vi "Configure.vi"(8 "error in (no error)":errorcluster, 11 "Switching Times in":refnum<class "Switching Time.lvclass">) -> (0 "error out":errorcluster, 3 "Switching Times out":refnum<class "Switching Time.lvclass">)   [LabVIEW 2020, in "Switching Time.lvclass"]
doc: "Configure the measurements paramaters to sweep.\nThis should be a pop up interface invoked by the configure test button on the main panel."
uses:
  Switching Time.lvclass
  Controls/Method.ctl
panel:
  in  "System Cancel Button":bool
  in  "Channels and optional channel names":cluster{"Enabled":bool, "Channel name":string}[](array[cluster])
  in  "Method":T1
  in  "OK Button":bool
  # "Please setup\noscilloscope\nmanually.\nE.g. vertical \nand horizontal \nrange, trigger etc."
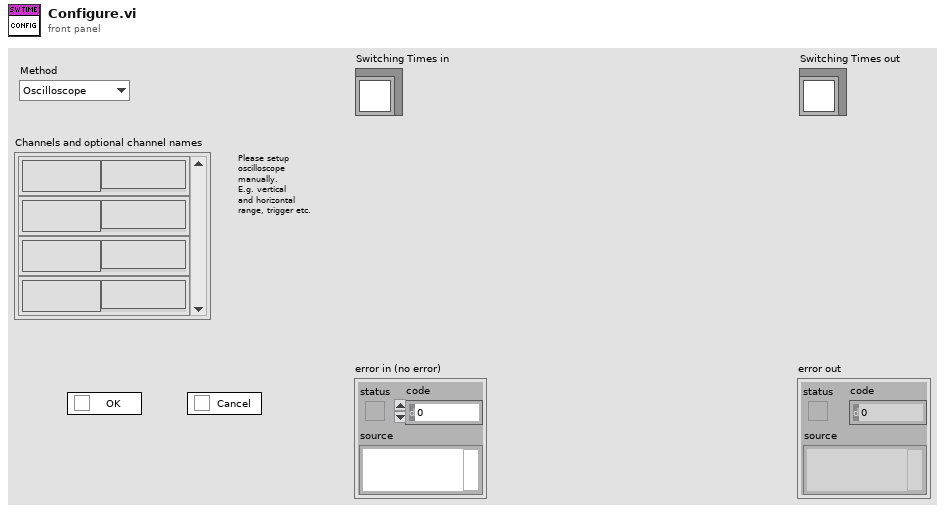
[diagram p1: front panel]
types:
  T1 = typedef "Switching Time.lvclass/Method.ctl" = enum16{"Oscilloscope", "Spectrum Analyzer"}
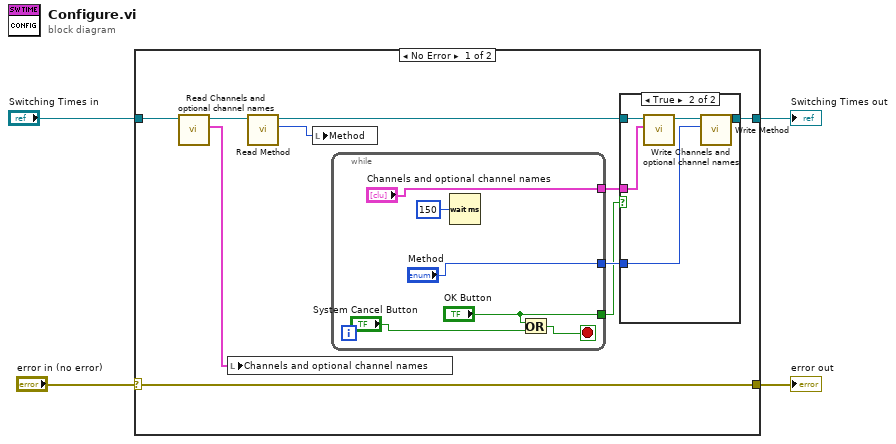
[diagram p0: block diagram]
diagram:
  n1 = case shown="No Error" "error in (no error)" {
    selector: "error in (no error)" -> [w12 w28]
    tunnel: "Switching Times in" -> [w9 w27]
    tunnel: [w14 w27] -> w2
    tunnel: [w12 w28] -> w1
    frame No Error {
      n2 = call-dynamic "Read Channels and optional channel names.vi"("Switching Time in"=w9) -> ("Channels and optional channel names"=w7:cluster{"Enabled":bool, "Channel name":string}[], "Switching Time out"=w10:refnum<class "Switching Time.lvclass">)  [unwired: 9 in]
      n3 = local write "Channels and optional channel names"(w7) -> ()
      n4 = call-dynamic "Read Method.vi"("Switching Time in"=w10) -> ("Method"=w6:T1, "Switching Time out"=w8:refnum<class "Switching Time.lvclass">)  [unwired: 9 in]
      n5 = local write "Method"(w6) -> ()
      n6 = while {
        tunnel: ["Method"] -> w13
        tunnel: ["Channels and optional channel names"] -> w11
        tunnel: ["OK Button"] -> w5
        stop <- w21 stop-if-true
        n7 = Wait (ms)(milliseconds to wait=u32 150) -> ()  [unwired: 1 out]
        n8 = Or(x="OK Button", y="System Cancel Button") -> (x .or. y?=w21:bool)
      }
      n9 = case shown="True" w5 {
        tunnel: [w15 w20] -> w14
        tunnel: w13 -> [_ w19]
        tunnel: w11 -> [_ w18]
        tunnel: w8 -> [w15 w16]
        frame False {
        }
        frame True {
          n10 = call-dynamic "Write Channels and optional channel names.vi"("Channels and optional channel names"=w18, "Switching Time in"=w16) -> ("Switching Time out"=w17:refnum<class "Switching Time.lvclass">)  [unwired: 9 in]
          n11 = call-dynamic "Write Method.vi"("Method"=w19, "Switching Time in"=w17) -> ("Switching Time out"=w20:refnum<class "Switching Time.lvclass">)  [unwired: 9 in]
        }
      }
    }
    frame Error {
    }
  }
  "error out" <- w1
  "Switching Times out" <- w2
